vi "get communication message.vi"(8 "error in (no error)":errorcluster, 11 "Channel in":refnum<class "Channel.lvclass">) -> (0 "error out":errorcluster, 3 "Channel out":refnum<class "Channel.lvclass">)   [LabVIEW 2018, in "Channel.lvclass"]
uses:
  Channel.lvclass
  Channel.lvclass/Channel.ctl
  RxTx/RxTx.lvclass
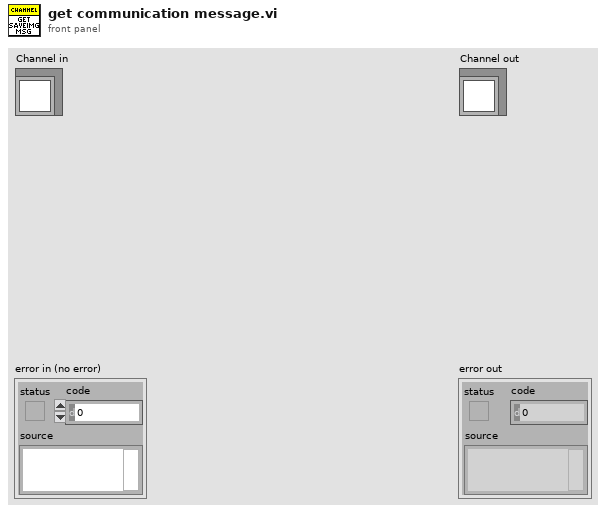
[diagram p1: front panel]
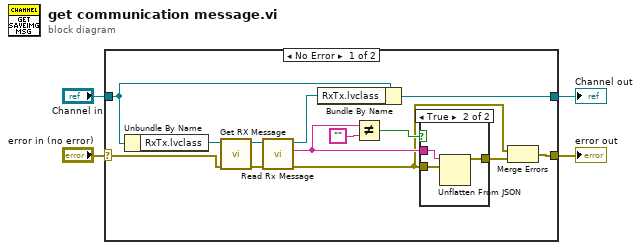
[diagram p0: block diagram]
diagram:
  n1 = case shown="No Error" "error in (no error)" {
    selector: "error in (no error)" -> [w12 w22]
    tunnel: [w10 w22] -> w3
    tunnel: [w16 w21] -> w1
    tunnel: "Channel in" -> [w17 w21]
    frame No Error {
      n2 = Unbundle By Name(w17) -> ("RxTx.lvclass"=w15:refnum<class "RxTx.lvclass">)
      n3 = call "Get RX Message.vi"("error in (no error)"=w12, "RxTx in"=w15) -> ("error out"=w11:errorcluster, "RxTx out"=w14:refnum<class "RxTx.lvclass">)  [unwired: 8 in]
      n4 = call "Read Rx Message.vi"("error in (no error)"=w11, "RxTx in"=w14) -> ("error out"=w5:errorcluster, "Rx Message"=w8:string, "RxTx out"=w13:refnum<class "RxTx.lvclass">)  [unwired: 7 in]
      n5 = Bundle By Name(cluster=w17, "RxTx.lvclass"=w13) -> (w16:refnum<class "Channel.lvclass">)
      n6 = Not Equal?(x=w8, y="") -> (x != y?=w7:bool)
      n7 = case shown="True" w7 {
        tunnel: w5 -> [_ w20]
        tunnel: w8 -> [_ w19]
        tunnel: [_ w18] -> w9
        frame False {
        }
        frame True {
          n8 = Unflatten From JSON(JSON string=w19, type and defaults=w20) -> (value=w18:errorcluster)  [unwired: 5 in, 1 out]
        }
      }
      n9 = Merge Errors(w5, w9) -> (w10:errorcluster)
    }
    frame Error {
    }
  }
  "error out" <- w3
  "Channel out" <- w1
